vi "sub build bp data.vi"(8 "error in":errorcluster, 11 "<bp> data":T1) -> (0 "error out":errorcluster, 3 "<bp> string":string)   [LabVIEW 2018, in "Data Parser.lvclass"]
uses:
  Data Parser.lvclass
  frame bp data.ctl
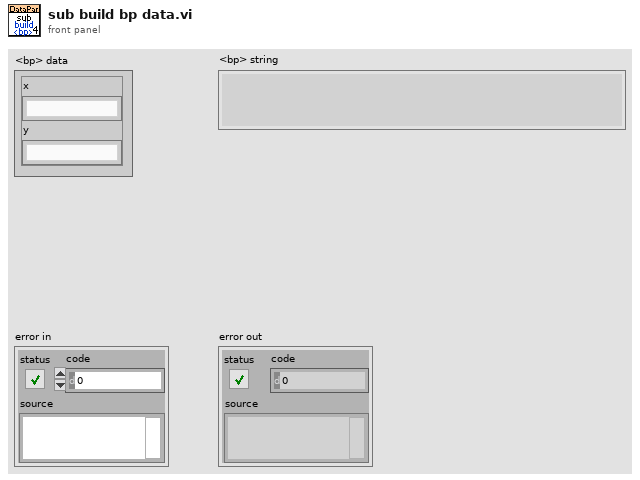
[diagram p1: front panel]
types:
  T1 = typedef "Data Parser.lvclass/frame bp data.ctl" = cluster{"x":string, "y":string}
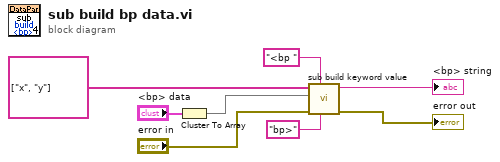
[diagram p0: block diagram]
diagram:
  n1 = Cluster To Array(cluster="<bp> data") -> (array=w6:string[])
  n2 = call "sub build keyword value.vi"("EOF"="bp>" ("SOF"), "SOF"="<bp ", "error in"="error in", "value"=w6, "keyword"=string[] ["x", "y"]) -> ("error out"=→"error out":errorcluster, "keyword value string"=→"<bp> string":string)  [unwired: 5 in]
